vi "SMSread.vi"(0 "HULK SMS address in":refnum<visa-resource-name>, 2 "SMS controls":T1, 5 "error in":errorcluster) -> (14 "HULK SMS address out":refnum<visa-resource-name>, 15 "read totally":u32, 16 "read buffer":string, 17 "Iterations":i32, 18 "after read":u32, 19 "error out":errorcluster)   [LabVIEW 2021]
uses:
  SMScontrols.ctl
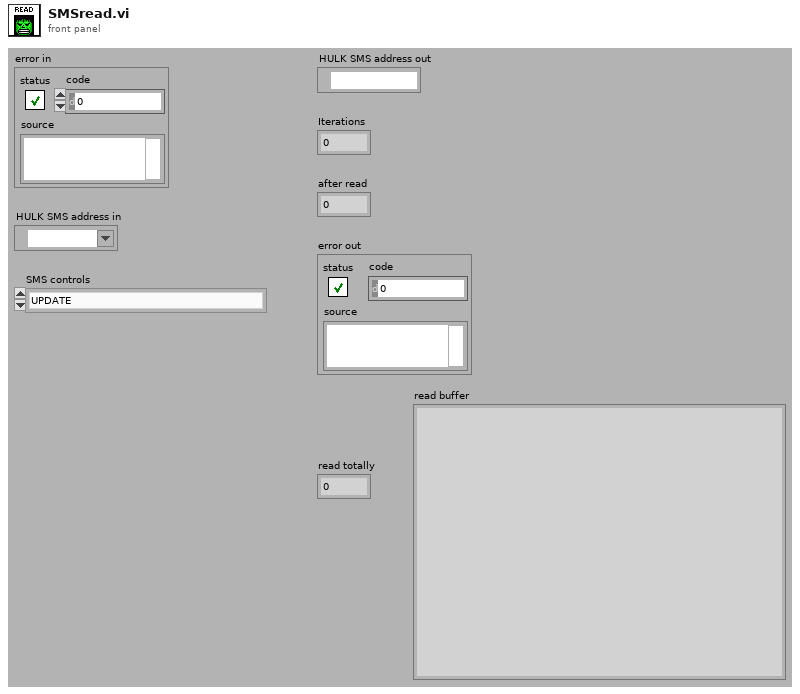
[diagram p1: front panel]
types:
  T1 = typedef "SMScontrols.ctl" = enum16{"UPDATE", "GET OUTPUT", "RAMP ZERO", "RAMP MID", "RAMP MAX", "RAMP STATUS", "PAUSE OFF", "PAUSE ON", "HEATER OFF", "HEATER ON", "TESLA OFF", "TESLA ON", "DIRECTION +", "DIRECTION -", "DIRECTION 0", "SET MID", "SET MAX", "SET RAMP", "SET LIMIT", "SET TPA", "SET HEATER"}
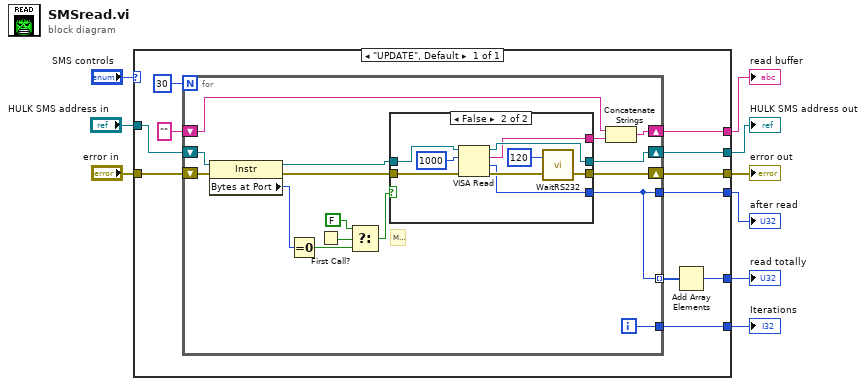
[diagram p0: block diagram]
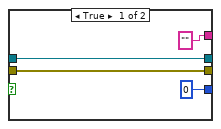
[diagram p2: hidden frame]
diagram:
  # "Missing object. The object \"Loop Condition\" does not exist in the previous version."
  n1 = case shown="\"UPDATE\", Default" "SMS controls" {
    tunnel: "HULK SMS address in" -> [w17]
    tunnel: "error in" -> [w16]
    tunnel: [w19] -> w5
    tunnel: [w18] -> w6
    tunnel: [w20] -> w3
    tunnel: [w12] -> w7
    tunnel: [w11] -> w8
    tunnel: [w10] -> w9
    frame "UPDATE", Default {
      n2 = for {
        N: 30 ("Numeric") -> [_]
        shift-right: [w33] -> w20
        shift-left: "" ("read buffer") -> [w35]
        shift-right: [w32] -> w18
        shift-left: w16 -> [w27]
        shift-right: [w36] -> w19
        shift-left: w17 -> [w28]
        tunnel: [w22] -> w13 mode=indexing
        tunnel: [w22] -> w11
        tunnel: [w31] -> w10
        i -> [w31]
        n3 = property class="Instr"(reference=w28, error in=w27) -> (reference out=w26:refnum<visa-resource-name>, error out=w25:errorcluster, "Bytes at Port"=w23:u32)
        n4 = Equal To 0?(x=w23) -> (x = 0?=w24:bool)
        n5 = First Call?() -> (First Call?: T/F=w30:bool)
        n6 = Select(t=FALSE, s=w30, f=w24) -> (s? t:f=w21:bool)
        n7 = case shown="False" w21 {
          tunnel: [w39 w49] -> w36
          tunnel: ["" ("read buffer") w48] -> w34
          tunnel: [w38 w46] -> w32
          tunnel: w26 -> [w39 w43]
          tunnel: w25 -> [w38 w42]
          tunnel: [u32 0 ("return count") w41] -> w22
          frame True {
          }
          frame False {
            n8 = VISA Read(VISA resource name=w43, byte count=u32 1000, error in (no error)=w42) -> (VISA resource name out=w49:refnum<visa-resource-name>, read buffer=w48:string, return count=w41:u32, error out=w47:errorcluster)
            n9 = call "WaitRS232.vi"("error in"=w47, "delay[160 ms]"=u32 120) -> ("error out"=w46:errorcluster)  [unwired: 1 in]
          }
        }
        n10 = Concatenate Strings(w35, w34) -> (w33:string)
      }
      n11 = Add Array Elements(numeric array=w13) -> (sum=w12:u32)
    }
  }
  "Iterations" <- w9
  "after read" <- w8
  "read totally" <- w7
  "error out" <- w6
  "HULK SMS address out" <- w5
  "read buffer" <- w3
